vi "Set Device Baud Rate.vi"(8 "error in (no error)":errorcluster, 10 "Baud Rate":u32=9600, 11 "Handle":u64) -> (0 "error out":errorcluster, 3 "Handle out":u64)   [LabVIEW 2019, in "D2XX-lv.lvlib"]
doc: "This function sets the baud rate for an open device."
uses:
  D2XX-lv.lvlib
  <instrlib>/_D2XX/D2XX/D2XX.lvlib
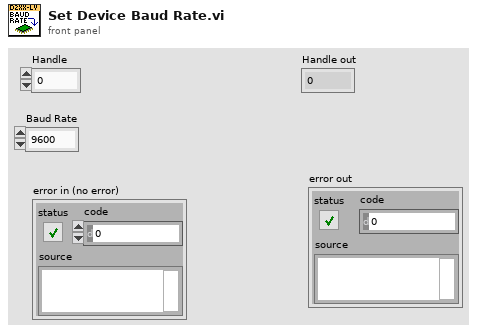
[diagram p1: front panel]
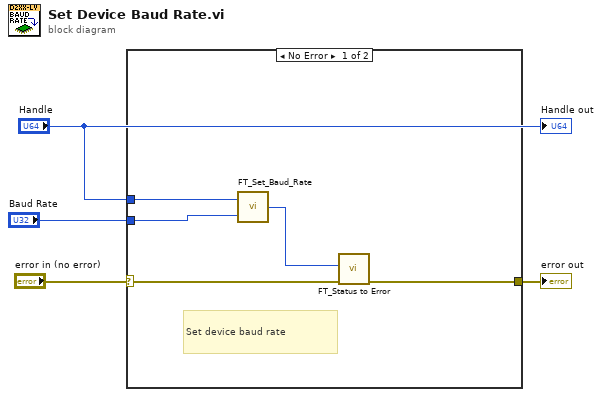
[diagram p0: block diagram]
diagram:
  n1 = case shown="No Error" "error in (no error)" {
    selector: "error in (no error)" -> [w9 w10]
    tunnel: [w5 w10] -> w3
    tunnel: "Handle" -> [w7 _]
    tunnel: "Baud Rate" -> [w6 _]
    frame No Error {
      # "Set device baud rate"
      n2 = call <instrlib>:"FT_Set_Baud_Rate.vi"("Baud Rate"=w6, "Handle"=w7) -> ("FT_Status"=w8:u32)
      n3 = call "FT_Status to Error.vi"("error in (no error)"=w9, "FT_Status"=w8) -> ("error out"=w5:errorcluster)  [unwired: 9 in]
    }
    frame Error {
    }
  }
  "error out" <- w3
  "Handle out" <- "Handle"
